vi "init.vi"(8 "error in (no error)":errorcluster, 11 "FlowControlValveCompensator in":refnum<class "FlowControlValveCompensator.lvclass">) -> (0 "error out":errorcluster, 3 "FlowControlValveCompensator out":refnum<class "FlowControlValveCompensator.lvclass">)   [LabVIEW 2013, in "FlowControlValveCompensator.lvclass"]
uses:
  FlowControlValveCompensator.lvclass
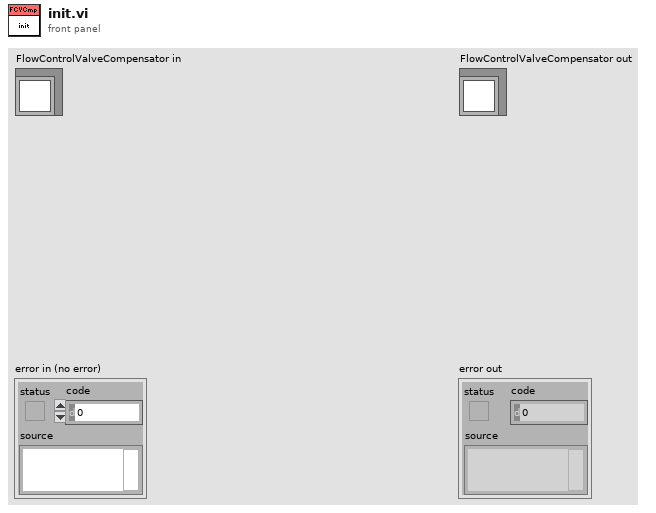
[diagram p1: front panel]
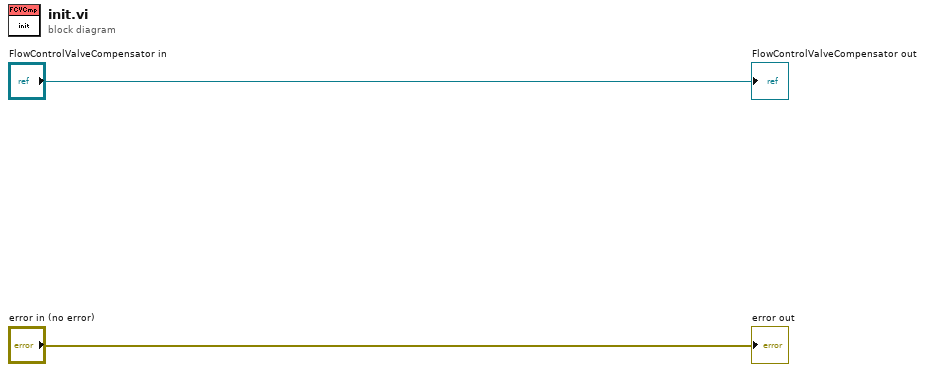
[diagram p0: block diagram]
diagram:
  "error out" <- "error in (no error)"
  "FlowControlValveCompensator out" <- "FlowControlValveCompensator in"
